vi "9048_Counter.vi"() -> ()   [LabVIEW 2023]
panel:
  out "Val":i32
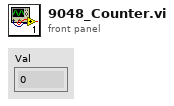
[diagram p1: front panel]
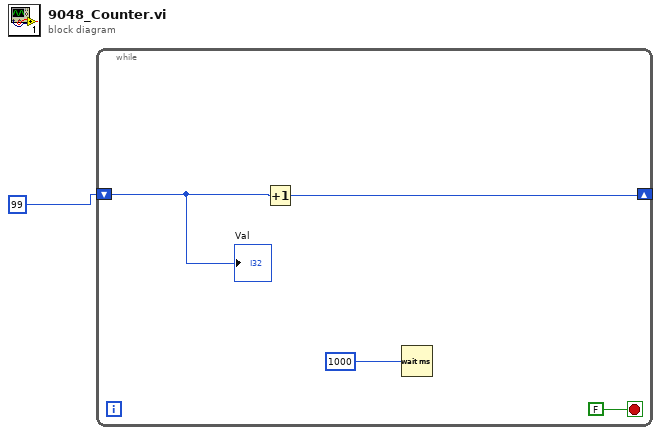
[diagram p0: block diagram]
diagram:
  n1 = while {
    shift-right: [w4] -> _
    shift-left: 99 -> [w3]
    stop <- FALSE stop-if-true
    n2 = Increment(x=w3) -> (x+1=w4:i32)
    n3 = Wait (ms)(milliseconds to wait=u32 1000) -> ()  [unwired: 1 out]
    "Val" <- w3
  }
